vi "Heater Control.vi"() -> ()   [LabVIEW 2017]
uses:
  <vilib>/Utility/error.llb/Clear Errors.vi
  <instrlib>/tio-labview/TIO Library/TIO RPC Send REQuest.vi
  <instrlib>/tio-labview/TIO Library/TIO RPC Parse Reply.vi
  <instrlib>/tio-labview/TIO Library/TIO RPC Parse Reply Error.vi
  <instrlib>/tio-labview/TIO Library/TIO Data Stream Parse timebase Info.vi
  <instrlib>/tio-labview/TIO Library/TIO Data Stream Parse pstream Info.vi
  <instrlib>/tio-labview/TIO Library/TIO Data Stream Parse dstream Info.vi
  <instrlib>/tio-labview/TIO Library/TIO Stream Write.vi
  <instrlib>/tio-labview/TIO Library/TIO RPC Form Request.vi
  <instrlib>/tio-labview/TIO Library/TIO SLIP Serial Write.vi
  <instrlib>/tio-labview/TIO Library/TIO Form Packet.vi
  <instrlib>/tio-labview/TIO Library/TIO SLIP Encode.vi
  <instrlib>/tio-labview/TIO Library/TIO Serial Checksum CRC32.vi
  <instrlib>/tio-labview/TIO Library/TIO Stream Read Non-blocking.vi
panel:
  in  "prefix":string="therm"
  in  "Voltage Max":dbl[unit] format="%#_4g"
  in  "Voltage Full Scale":dbl[unit] format="%#_4g"
  in  "Voltage":dbl[unit] format="%#_4g"
  in  "Manual":bool
  in  "Freq":dbl[unit] format="%#_4g"
  in  "Autostart":bool
  in  "Ki":dbl format="%#_4g"
  in  "Kp":dbl format="%#_4g"
  out "Resistance Measured":dbl[unit] format="%#_4g"
  in  "Save":bool
  in  "Calibrate R0":bool
  in  "Load":dbl[unit] format="%#_4g"
  in  "Heater Enable":bool
  out "Power Output":dbl[unit] format="%#_4f"
  in  "Power Max":dbl[unit] format="%#_4f"
  out "Temperature Measured":dbl[unit] format="%#_4g"
  in  "Temperature Set":dbl[unit] format="%#_4g"
  in  "URL":refnum<visa-resource-name>="tcp://localhost"
  out "ID":string
  in  "Quit":bool
  in  "Duration":dbl[unit]=1000.0
  in  "Reset":bool
  out "Temperature":T1(graph)
  # "Heater"
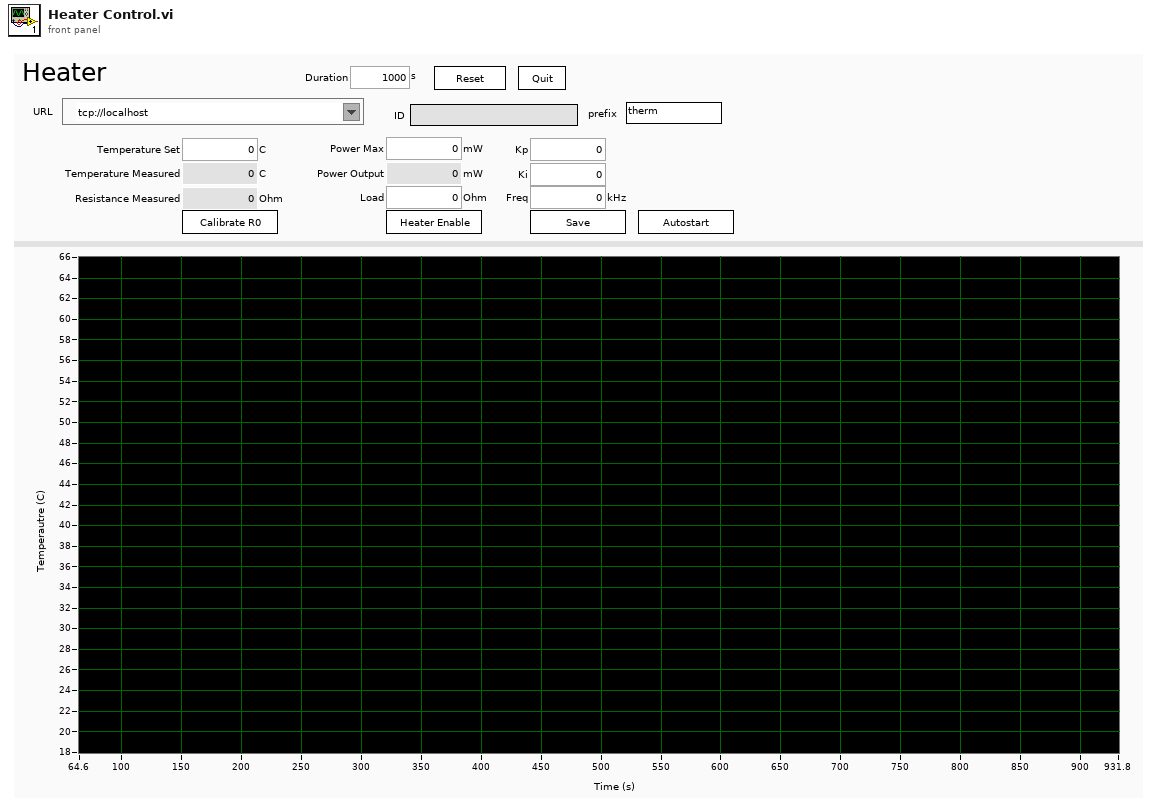
[diagram p1: front panel]
types:
  T1 = cluster{"start":dbl, "dt":dbl, "Timeseries":dbl[]}
  T2 = cluster{"TS Connection":cluster{"Type":enum16{"TCP", "Serial"}, "Serial":refnum<visa-resource-name>, "TCP":refnum<k5>, "Timeout":u32}, "REQ":refnum<queue>, "REP":refnum<queue>}
  T3 = cluster{"Awaiting REP":bool, "REQ ID":u32, "dstreams in":cluster{"id":u16, "timebase id":u16, "period":u32, "offset":u32, "sample number":u64, "total components":u16, "flags":u16, "components":cluster{"pstream id":u16, "flags":u16, "period":u32, "offset":u32}[]}[], "pstreams":cluster{"id":u16, "timebase_id":u16, "period":u32, "offset":u32, "fmt":i32, "flags":u16, "channels":u16, "type":u8, "name":string, "column names":string[], "title":string, "units":string}[], "timebases":cluster{"id":u16, "source":u16, "epoch":u32, "start time":u32, "period numerator (µs)":i32, "period denominator (µs)":u16, "flags":u16, "stability":u8, "source id":string}[]}
  T4 = cluster{"dstream ID":u16, "Sample Number":u32, "Raw Data":string}
  T5 = cluster{"Name":string, "Waveform":cluster{"start":dbl, "dt":dbl, "Timeseries":dbl[][]}}[]
  T6 = cluster{"start":dbl, "dt":dbl, "Timeseries":dbl[][]}
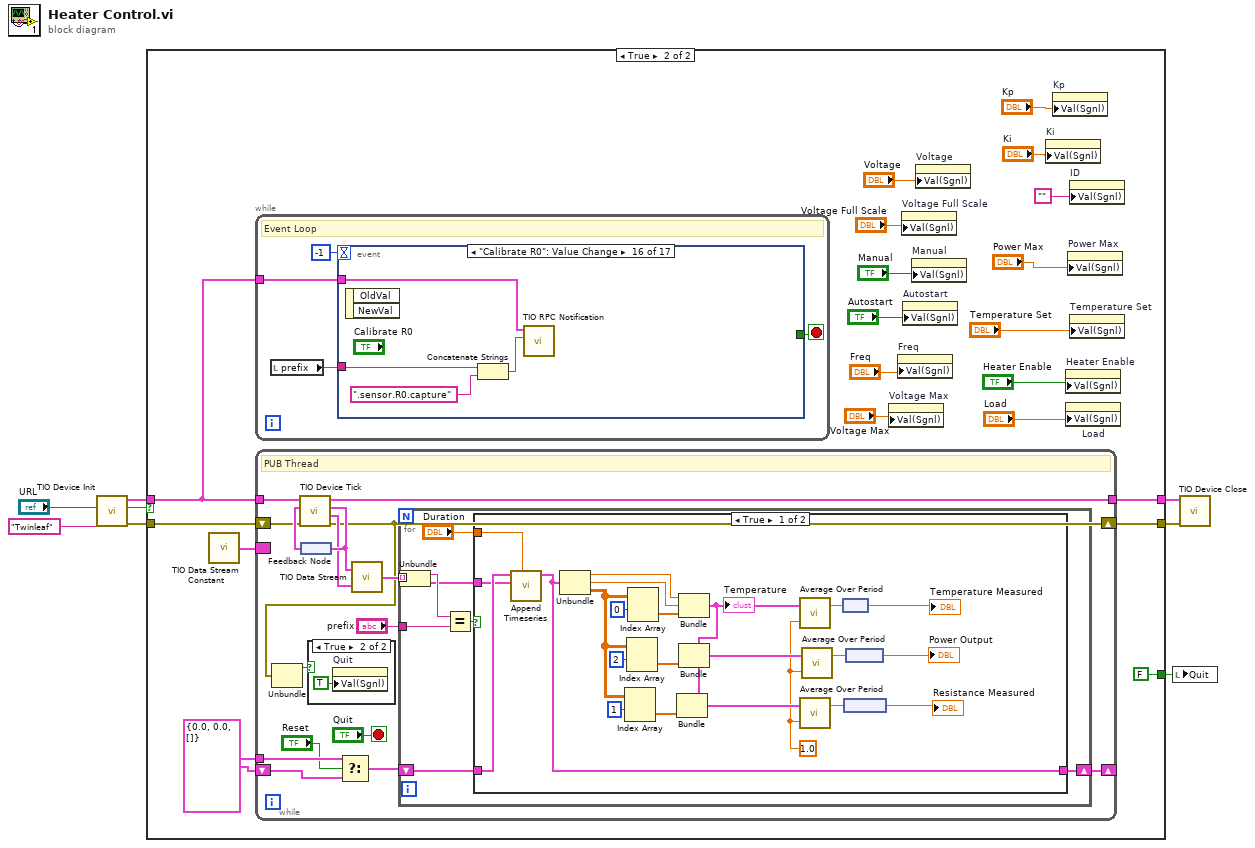
[diagram p0: block diagram]
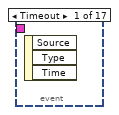
[diagram p5: hidden frame]
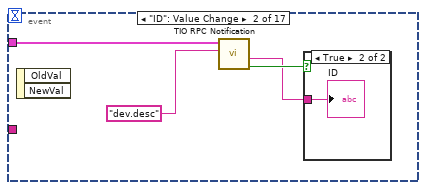
[diagram p6: hidden frame]
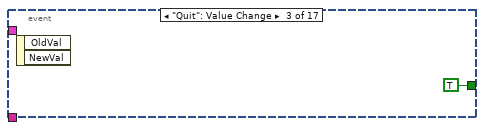
[diagram p8: hidden frame]
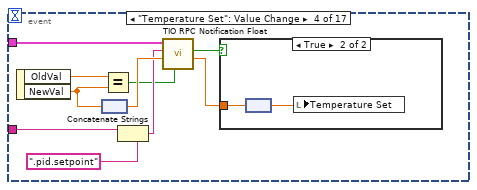
[diagram p9: hidden frame]
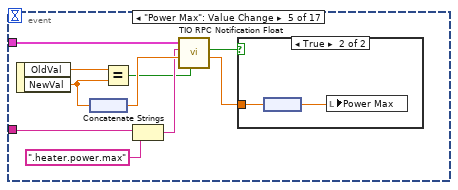
[diagram p11: hidden frame]
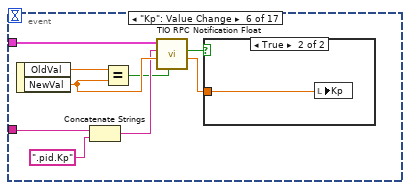
[diagram p13: hidden frame]
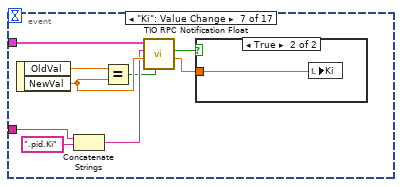
[diagram p15: hidden frame]
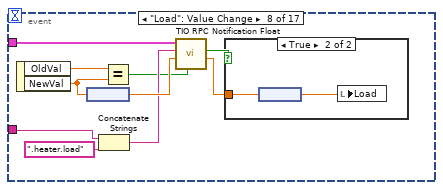
[diagram p17: hidden frame]
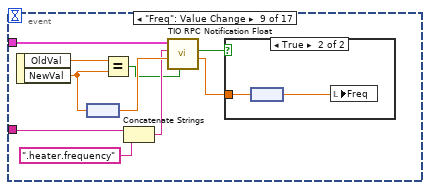
[diagram p19: hidden frame]
diagram:
  n1 = call <instrlib>:"TIO Device Init.vi"("ID"="Twinleaf", "URL"="URL") -> ("error out"=w4:errorcluster, "ID Verified"=w5:bool, "TIO"=w6:T2)  [unwired: 6 in, 1 out]
  n2 = case shown="True" w5 {
    tunnel: w6 -> [w10 w15]
    tunnel: w4 -> [w9 w16]
    tunnel: [_ FALSE ("Quit")] -> w3
    tunnel: [w10 w12] -> w2
    tunnel: [w9 w11] -> w1
    frame False {
    }
    frame True {
      w13 = cluster{dbl, dbl, dbl[][]} {0.0, 0.0, []} ("Waveform Timeseries")
      n3 = call <instrlib>:"TIO Data Stream Constant.vi"() -> ("TIO State"=w17:T3)
      n4 = while {
        tunnel: w15 -> [w82]
        stop <- w80 stop-if-true
        # "Event Loop"
        n5 = local read "prefix"() -> (w81:string)
        n6 = event shown="[15] \"Calibrate R0\": Value Change" {
          selector: _ -> [_ _ _ _ _ _ _ _ _ _ _ _ _ _ _ _ _]
          dyn-events: _ -> [_ _ _ _ _ _ _ _ _ _ _ _ _ _ _ _ _]
          timeout: -1 -> [_ _ _ _ _ _ _ _ _ _ _ _ _ _ _ _ _]
          tunnel: w81 -> [_ _ _ w93 w106 w118 w127 w138 w149 w161 w174 w186 w198 w209 w222 w233 _]
          tunnel: w82 -> [_ w84 _ w92 w104 w116 w124 w136 w147 w159 w172 w183 w195 w208 w219 w231 w235]
          tunnel: [_ _ TRUE ("Quit") _ _ _ _ _ _ _ _ _ _ _ _ _ _] -> w80
          event Timeout {
            n7 = event-data() -> ()  [unwired: 1 in, 3 out]
          }
          event "ID": Value Change {
            n8 = event-data() -> ()  [unwired: 1 in, 2 out]
            n9 = call <instrlib>:"TIO RPC Notification.vi"("Topic"="dev.desc", "TIO"=w84) -> ("REP"=w86:string, "Response"=w87:bool)  [unwired: 6 in, 1 out]
            n10 = case shown="True" w87 {
              tunnel: w86 -> [_ w88]
              frame False {
              }
              frame True {
                "ID" <- w88
              }
            }
          }
          event "Quit": Value Change {
            n11 = event-data() -> ()  [unwired: 1 in, 2 out]
          }
          event "Temperature Set": Value Change {
            n12 = event-data() -> ("OldVal"=w99:dbl[unit], "NewVal"=w95:dbl[unit])  [unwired: 1 in]
            n13 = node(w95) -> (w98:dbl)
            n14 = Equal?(x=w99, y=w95) -> (x = y?=w90:bool)
            n15 = Concatenate Strings(w93, ".pid.setpoint" ("String")) -> (w91:string)
            n16 = call <instrlib>:"TIO RPC Notification Float.vi"("Read"=w90, "Set value"=w98, "Topic"=w91, "TIO"=w92) -> ("Get value (default if error)"=w96:sgl, "Response"=w97:bool)  [unwired: 4 in, 1 out]
            n17 = case shown="True" w97 {
              tunnel: w96 -> [_ w101]
              frame False {
              }
              frame True {
                n18 = node(w101) -> (w100:sgl[unit])
                n19 = local write "Temperature Set"(w100) -> ()
              }
            }
          }
          event "Power Max": Value Change {
            n20 = event-data() -> ("OldVal"=w111:dbl[unit], "NewVal"=w107:dbl[unit])  [unwired: 1 in]
            n21 = node(w107) -> (w110:dbl)
            n22 = Equal?(x=w111, y=w107) -> (x = y?=w102:bool)
            n23 = Concatenate Strings(w106, ".heater.power.max" ("String")) -> (w103:string)
            n24 = call <instrlib>:"TIO RPC Notification Float.vi"("Read"=w102, "Set value"=w110, "Topic"=w103, "TIO"=w104) -> ("Get value (default if error)"=w108:sgl, "Response"=w109:bool)  [unwired: 4 in, 1 out]
            n25 = case shown="True" w109 {
              tunnel: w108 -> [_ w113]
              frame False {
              }
              frame True {
                n26 = node(w113) -> (w112:sgl[unit])
                n27 = local write "Power Max"(w112) -> ()
              }
            }
          }
          event "Kp": Value Change {
            n28 = event-data() -> ("OldVal"=w122:dbl, "NewVal"=w119:dbl)  [unwired: 1 in]
            n29 = Concatenate Strings(w118, ".pid.Kp" ("String")) -> (w115:string)
            n30 = Equal?(x=w122, y=w119) -> (x = y?=w114:bool)
            n31 = call <instrlib>:"TIO RPC Notification Float.vi"("Read"=w114, "Set value"=w119, "Topic"=w115, "TIO"=w116) -> ("Get value (default if error)"=w120:sgl, "Response"=w121:bool)  [unwired: 4 in, 1 out]
            n32 = case shown="True" w121 {
              tunnel: w120 -> [_ w123]
              frame False {
              }
              frame True {
                n33 = local write "Kp"(w123) -> ()
              }
            }
          }
          event "Ki": Value Change {
            n34 = event-data() -> ("OldVal"=w132:dbl, "NewVal"=w129:dbl)  [unwired: 1 in]
            n35 = Concatenate Strings(w127, ".pid.Ki" ("String")) -> (w126:string)
            n36 = Equal?(x=w132, y=w129) -> (x = y?=w125:bool)
            n37 = call <instrlib>:"TIO RPC Notification Float.vi"("Read"=w125, "Set value"=w129, "Topic"=w126, "TIO"=w124) -> ("Get value (default if error)"=w130:sgl, "Response"=w131:bool)  [unwired: 4 in, 1 out]
            n38 = case shown="True" w131 {
              tunnel: w130 -> [_ w133]
              frame False {
              }
              frame True {
                n39 = local write "Ki"(w133) -> ()
              }
            }
          }
          event "Load": Value Change {
            n40 = event-data() -> ("OldVal"=w143:dbl[unit], "NewVal"=w139:dbl[unit])  [unwired: 1 in]
            n41 = node(w139) -> (w142:dbl)
            n42 = Concatenate Strings(w138, ".heater.load" ("String")) -> (w135:string)
            n43 = Equal?(x=w143, y=w139) -> (x = y?=w134:bool)
            n44 = call <instrlib>:"TIO RPC Notification Float.vi"("Read"=w134, "Set value"=w142, "Topic"=w135, "TIO"=w136) -> ("Get value (default if error)"=w140:sgl, "Response"=w141:bool)  [unwired: 4 in, 1 out]
            n45 = case shown="True" w141 {
              tunnel: w140 -> [_ w145]
              frame False {
              }
              frame True {
                n46 = node(w145) -> (w144:sgl[unit])
                n47 = local write "Load"(w144) -> ()
              }
            }
          }
          event "Freq": Value Change {
            n48 = event-data() -> ("OldVal"=w155:dbl[unit], "NewVal"=w151:dbl[unit])  [unwired: 1 in]
            n49 = node(w151) -> (w154:dbl)
            n50 = Equal?(x=w155, y=w151) -> (x = y?=w146:bool)
            n51 = Concatenate Strings(w149, ".heater.frequency" ("String")) -> (w148:string)
            n52 = call <instrlib>:"TIO RPC Notification Float.vi"("Read"=w146, "Set value"=w154, "Topic"=w148, "TIO"=w147) -> ("Get value (default if error)"=w152:sgl, "Response"=w153:bool)  [unwired: 4 in, 1 out]
            n53 = case shown="True" w153 {
              tunnel: w152 -> [_ w157]
              frame False {
              }
              frame True {
                n54 = node(w157) -> (w156:sgl[unit])
                n55 = local write "Freq"(w156) -> ()
              }
            }
          }
          event "Voltage": Value Change {
            n56 = event-data() -> ("OldVal"=w167:dbl[unit], "NewVal"=w163:dbl[unit])  [unwired: 1 in]
            n57 = node(w163) -> (w166:dbl)
            n58 = Equal?(x=w167, y=w163) -> (x = y?=w158:bool)
            n59 = Concatenate Strings(w161, ".heater.amplitude" ("String")) -> (w160:string)
            n60 = call <instrlib>:"TIO RPC Notification Float.vi"("Read"=w158, "Set value"=w166, "Topic"=w160, "TIO"=w159) -> ("Get value (default if error)"=w164:sgl, "Response"=w165:bool)  [unwired: 4 in, 1 out]
            n61 = case shown="True" w165 {
              tunnel: w164 -> [_ w169]
              frame False {
              }
              frame True {
                n62 = node(w169) -> (w168:sgl[unit])
                n63 = local write "Voltage"(w168) -> ()
              }
            }
          }
          event "Voltage Max": Value Change {
            n64 = event-data() -> ("OldVal"=w179:dbl[unit], "NewVal"=w175:dbl[unit])  [unwired: 1 in]
            n65 = node(w175) -> (w178:dbl)
            n66 = Equal?(x=w179, y=w175) -> (x = y?=w171:bool)
            n67 = Concatenate Strings(w174, ".heater.amplitude.max" ("String")) -> (w170:string)
            n68 = call <instrlib>:"TIO RPC Notification Float.vi"("Read"=w171, "Set value"=w178, "Topic"=w170, "TIO"=w172) -> ("Get value (default if error)"=w176:sgl, "Response"=w177:bool)  [unwired: 4 in, 1 out]
            n69 = case shown="True" w177 {
              tunnel: w176 -> [_ w181]
              frame False {
              }
              frame True {
                n70 = node(w181) -> (w180:sgl[unit])
                n71 = local write "Voltage Max"(w180) -> ()
              }
            }
          }
          event "Voltage Full Scale": Value Change {
            n72 = event-data() -> ("OldVal"=w191:dbl[unit], "NewVal"=w187:dbl[unit])  [unwired: 1 in]
            n73 = node(w187) -> (w190:dbl)
            n74 = Equal?(x=w191, y=w187) -> (x = y?=w182:bool)
            n75 = Concatenate Strings(w186, ".heater.amplitude.scale" ("String")) -> (w184:string)
            n76 = call <instrlib>:"TIO RPC Notification Float.vi"("Read"=w182, "Set value"=w190, "Topic"=w184, "TIO"=w183) -> ("Get value (default if error)"=w188:sgl, "Response"=w189:bool)  [unwired: 4 in, 1 out]
            n77 = case shown="True" w189 {
              tunnel: w188 -> [_ w193]
              frame False {
              }
              frame True {
                n78 = node(w193) -> (w192:sgl[unit])
                n79 = local write "Voltage Full Scale"(w192) -> ()
              }
            }
          }
          event "Heater Enable": Value Change {
            n80 = event-data() -> ("OldVal"=w203:bool, "NewVal"=w199:bool)  [unwired: 1 in]
            n81 = Equal?(x=w203, y=w199) -> (x = y?=w194:bool)
            n82 = Boolean To (0,1)(Boolean=w199) -> (0, 1=w202:i16)
            n83 = Concatenate Strings(w198, ".pid.enable" ("String")) -> (w196:string)
            n84 = call <instrlib>:"TIO RPC Notification U8.vi"("Read"=w194, "U8"=w202, "Topic"=w196, "TIO"=w195) -> ("U8"=w200:u8, "Response"=w201:bool)  [unwired: 4 in, 1 out]
            n85 = case shown="True" w201 {
              tunnel: w200 -> [_ w205]
              frame False {
              }
              frame True {
                n86 = Greater Than 0?(x=w205) -> (x > 0?=w204:bool)
                n87 = local write "Heater Enable"(w204) -> ()
              }
            }
          }
          event "Autostart": Value Change {
            n88 = event-data() -> ("OldVal"=w215:bool, "NewVal"=w211:bool)  [unwired: 1 in]
            n89 = Equal?(x=w215, y=w211) -> (x = y?=w206:bool)
            n90 = Boolean To (0,1)(Boolean=w211) -> (0, 1=w214:i16)
            n91 = Concatenate Strings(w209, ".pid.autostart" ("String")) -> (w207:string)
            n92 = call <instrlib>:"TIO RPC Notification U8.vi"("Read"=w206, "U8"=w214, "Topic"=w207, "TIO"=w208) -> ("U8"=w212:u8, "Response"=w213:bool)  [unwired: 4 in, 1 out]
            n93 = case shown="True" w213 {
              tunnel: w212 -> [_ w217]
              frame False {
              }
              frame True {
                n94 = Greater Than 0?(x=w217) -> (x > 0?=w216:bool)
                n95 = local write "Autostart"(w216) -> ()
              }
            }
          }
          event "Manual": Value Change {
            n96 = event-data() -> ("OldVal"=w227:bool, "NewVal"=w223:bool)  [unwired: 1 in]
            n97 = Equal?(x=w227, y=w223) -> (x = y?=w220:bool)
            n98 = Boolean To (0,1)(Boolean=w223) -> (0, 1=w226:i16)
            n99 = Concatenate Strings(w222, ".pid.manual" ("String")) -> (w218:string)
            n100 = call <instrlib>:"TIO RPC Notification U8.vi"("Read"=w220, "U8"=w226, "Topic"=w218, "TIO"=w219) -> ("U8"=w224:u8, "Response"=w225:bool)  [unwired: 4 in, 1 out]
            n101 = case shown="True" w225 {
              tunnel: w224 -> [_ w229]
              frame False {
              }
              frame True {
                n102 = Greater Than 0?(x=w229) -> (x > 0?=w228:bool)
                n103 = local write "Manual"(w228) -> ()
              }
            }
          }
          event "Calibrate R0": Value Change {
            n104 = event-data() -> ()  [unwired: 1 in, 2 out]
            n105 = Concatenate Strings(w233, ".sensor.R0.capture" ("String")) -> (w230:string)
            n106 = call <instrlib>:"TIO RPC Notification.vi"("Topic"=w230, "TIO"=w231) -> ()  [unwired: 6 in, 3 out]
          }
          event "Save": Value Change {
            n107 = event-data() -> ()  [unwired: 1 in, 2 out]
            n108 = call <instrlib>:"TIO RPC Notification.vi"("Topic"="dev.conf.save" ("String"), "TIO"=w235) -> ()  [unwired: 6 in, 3 out]
          }
        }
      }
      n109 = while {
        shift-right: [w46] -> _
        shift-left: w13 -> [w37]
        border: w17 -> [_]
        tunnel: w15 -> [w42]
        tunnel: w13 -> [w35]
        tunnel: [w33] -> w12
        shift-right: [w32] -> w11
        shift-left: w16 -> [w41]
        stop <- "Quit" stop-if-true
        # "PUB Thread"
        n110 = feedback #1() -> (w45:T3)
        n111 = call <instrlib>:"TIO Device Tick.vi"("Error in"=w41, "TIO State"=w45, "TIO"=w42) -> ("Error out"=w32:errorcluster, "Data Out"=w43:T4, "TIO State"=w44:T3, "TIO Out"=w33:T2)  [unwired: 5 in]
        n112 = Unbundle(w32) -> ("status"=w31:bool)  [unwired: 2 out]
        n113 = feedback-in #1(w44) -> ()
        n114 = case shown="True" w31 {
          frame False {
          }
          frame True {
            n115 = property on="Quit" class="Bool (strict)"("Val(Sgnl)"=TRUE ("Value (Signaling)")) -> ()  [unwired: 2 in, 2 out]
          }
        }
        n116 = Select(t=w35, s="Reset", f=w37) -> (s? t:f=w36:cluster{dbl, dbl, dbl[][]})
        n117 = call <instrlib>:"TIO Data Stream.vi"("Raw Data"=w43, "TIO State"=w44) -> ("Data Out"=w40:T5)
        n118 = for {
          tunnel: "prefix" -> [w51]
          shift-right: [w54] -> w46
          shift-left: w36 -> [w52]
          tunnel: w40 -> [w50] mode=indexing
          n119 = Unbundle(w50) -> ("Name"=w49:string, "Waveform"=w48:T6)
          n120 = Equal?(x=w49, y=w51) -> (x = y?=w53:bool)
          n121 = case shown="True" w53 {
            tunnel: "Duration" -> [w78 _]
            tunnel: [w76 w79] -> w54
            tunnel: w52 -> [w75 w79]
            tunnel: w48 -> [w56 _]
            frame True {
              w58 = dbl[unit] 1.0 ("Period")
              n122 = call <instrlib>:"Append Timeseries.vi"("Duration"=w78, "In New"=w56, "In Old"=w75) -> ("Appended"=w76:T6)  [unwired: 8 in]
              n123 = Unbundle(w76) -> ("start"=w61:dbl, "dt"=w60:dbl, "Timeseries"=w62:dbl[][])
              n124 = Index Array(array=w62, index (row)=1 ("disabled index (col)")) -> (element=w64:dbl[])  [unwired: 1 in]
              n125 = Index Array(array=w62, index (row)=2 ("disabled index (col)")) -> (element=w70:dbl[])  [unwired: 1 in]
              n126 = Index Array(array=w62, index (row)=0 ("disabled index (col)")) -> (element=w74:dbl[])  [unwired: 1 in]
              n127 = Bundle("start"=w61, "dt"=w60, "Timeseries"=w74) -> (w57:T1)  [unwired: 1 in]
              "Temperature" <- w57
              n128 = Bundle(cluster=w57, "Timeseries"=w64) -> (w65:T1)  [unwired: 2 in]
              n129 = Bundle(cluster=w57, "Timeseries"=w70) -> (w69:T1)  [unwired: 2 in]
              n130 = call <instrlib>:"Average Over Period.vi"("Period"=w58, "Cluster"=w57) -> ("Average"=w73:dbl)  [unwired: 1 in]
              n131 = call <instrlib>:"Average Over Period.vi"("Period"=w58, "Cluster"=w65) -> ("Average"=w66:dbl)  [unwired: 1 in]
              n132 = call <instrlib>:"Average Over Period.vi"("Period"=w58, "Cluster"=w69) -> ("Average"=w68:dbl)  [unwired: 1 in]
              n133 = node(w73) -> (→"Temperature Measured":dbl[unit])
              n134 = node(w66) -> (→"Resistance Measured":dbl[unit])
              n135 = node(w68) -> (→"Power Output":dbl[unit])
            }
            frame False {
            }
          }
        }
      }
      n136 = property on="Voltage Max" class="DigNum (strict)"("Val(Sgnl)"="Voltage Max") -> ()  [unwired: 2 in, 2 out]
      n137 = property on="Freq" class="DigNum (strict)"("Val(Sgnl)"="Freq") -> ()  [unwired: 2 in, 2 out]
      n138 = property on="Voltage Full Scale" class="DigNum (strict)"("Val(Sgnl)"="Voltage Full Scale") -> ()  [unwired: 2 in, 2 out]
      n139 = property on="Autostart" class="Bool (strict)"("Val(Sgnl)"="Autostart") -> ()  [unwired: 2 in, 2 out]
      n140 = property on="Manual" class="Bool (strict)"("Val(Sgnl)"="Manual") -> ()  [unwired: 2 in, 2 out]
      n141 = property on="Voltage" class="DigNum (strict)"("Val(Sgnl)"="Voltage") -> ()  [unwired: 2 in, 2 out]
      n142 = property on="Ki" class="DigNum (strict)"("Val(Sgnl)"="Ki") -> ()  [unwired: 2 in, 2 out]
      n143 = property on="Kp" class="DigNum (strict)"("Val(Sgnl)"="Kp") -> ()  [unwired: 2 in, 2 out]
      n144 = property on="Heater Enable" class="Bool (strict)"("Val(Sgnl)"="Heater Enable") -> ()  [unwired: 2 in, 2 out]
      n145 = property on="Load" class="DigNum (strict)"("Val(Sgnl)"="Load") -> ()  [unwired: 2 in, 2 out]
      n146 = property on="Power Max" class="DigNum (strict)"("Val(Sgnl)"="Power Max") -> ()  [unwired: 2 in, 2 out]
      n147 = property on="ID" class="Str"("Val(Sgnl)"="") -> ()  [unwired: 2 in, 2 out]
      n148 = property on="Temperature Set" class="DigNum (strict)"("Val(Sgnl)"="Temperature Set") -> ()  [unwired: 2 in, 2 out]
    }
  }
  n149 = local write "Quit"(w3) -> ()
  n150 = call <instrlib>:"TIO Device Close.vi"("Error in"=w1, "TIO"=w2) -> ()  [unwired: 10 in]
